vi "removeNode2.vi"(0 "reference":refnum<class "Graph.lvclass">, 1 "node":refnum<class "AbstractNode.lvclass">, 5 "error in (no error)":errorcluster) -> (14 "reference out":refnum<class "Graph.lvclass">, 19 "error out":errorcluster)   [LabVIEW 2016, in "Graph.lvclass"]
uses:
  <resource>/Framework/Providers/Open_GDS/UML/Graph_class/Graph.lvclass
  <resource>/Framework/Providers/Open_GDS/UML/AbstractNode_class/AbstractNode.lvclass
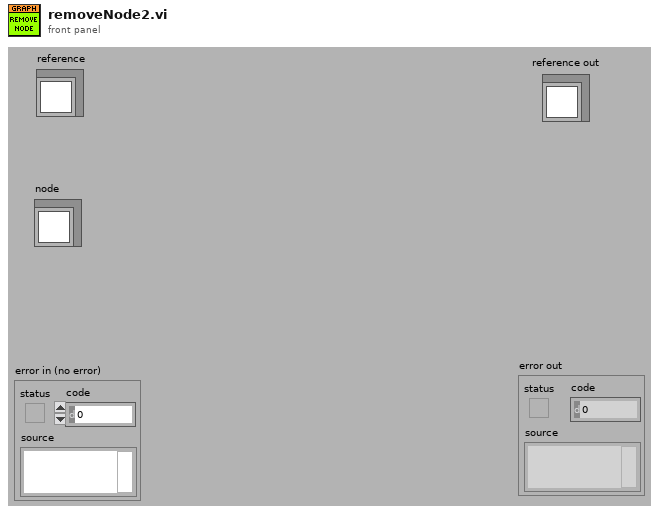
[diagram p1: front panel]
types:
  T1 = typedef "Graph.lvclass/ObjectAttributes.ctl" = cluster{"nodes":refnum<class "AbstractNode.lvclass">[], "edges":refnum<class "AbstractEdge.lvclass">[], "nodesToBeRemoved":refnum<class "AbstractNode.lvclass">[], "edgesToBeRemoved":refnum<class "AbstractEdge.lvclass">[], "needsLayout":bool, "LayoutNodes":refnum<class "AbstractNode.lvclass">[]}
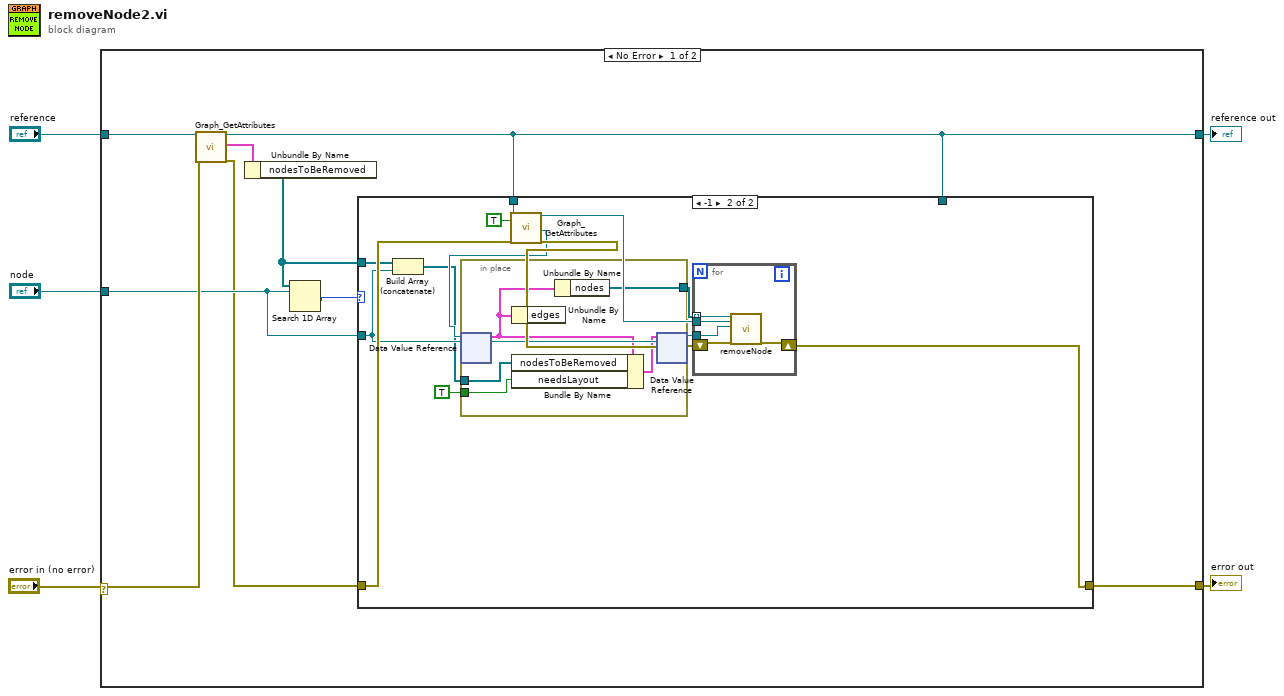
[diagram p0: block diagram]
diagram:
  n1 = case shown="No Error" "error in (no error)" {
    selector: "error in (no error)" -> [w11 w38]
    tunnel: "reference" -> [w14 w39]
    tunnel: [w13 w38] -> w4
    tunnel: [w12 w39] -> w3
    tunnel: "node" -> [w10 _]
    frame No Error {
      n2 = call <resource>:"Graph_GetAttributes.vi"("reference in"=w14, "error in (no error)"=w11) -> ("reference out"=w12:refnum<class "Graph.lvclass">, "Data"=w6:T1, "error out"=w8:errorcluster)  [unwired: 1 in, 14 out]
      n3 = Unbundle By Name(w6) -> ("nodesToBeRemoved"=w7:refnum<class "AbstractNode.lvclass">[])
      n4 = Search 1D Array(1D array=w7, element=w10) -> (index of element=w9:i32)  [unwired: 1 out]
      n5 = case shown="-1" w9 {
        tunnel: w8 -> [w15 w26]
        tunnel: [w15 w21] -> w13
        tunnel: w12 -> [_ w27]
        tunnel: w7 -> [_ w25]
        tunnel: w10 -> [_ w22]
        tunnel: w12 -> [_ _]
        frame 0, Default {
        }
        frame -1 {
          n6 = Build Array (concatenate)(w25, w22) -> (w17:refnum<class "AbstractNode.lvclass">[])
          n7 = call <resource>:"Graph_GetAttributes.vi"("reference in"=w27, "OnlyGetDvrReference(False)"=TRUE, "error in (no error)"=w26) -> ("reference out"=w24:refnum<class "Graph.lvclass">, "DataRef"=w19:refnum<data-value>, "error out"=w23:errorcluster)  [unwired: 13 in, 1 out]
          n8 = in-place {
            in-place-border: [w31] -> w18
            in-place-border: w17 -> [w30]
            in-place-border: TRUE ("needsLayout") -> [w29]
            n9 = in-place-dvr #1(w19) -> (w32:T1)  [unwired: 1 out]
            n10 = Unbundle By Name(w32) -> ()  [unwired: 1 out]
            n11 = Bundle By Name(cluster=w32, "nodesToBeRemoved"=w30, "needsLayout"=w29) -> (w28:T1)
            n12 = Unbundle By Name(w32) -> ("nodes"=w31:refnum<class "AbstractNode.lvclass">[])
            n13 = in-place-dvr #1(w28) -> ()  [unwired: 2 out]
          }
          n14 = for {
            tunnel: w18 -> [w37] mode=indexing
            tunnel: w24 -> [w36]
            tunnel: w22 -> [w35]
            shift-right: [w33] -> w21
            shift-left: w23 -> [w34]
            n15 = call-dynamic "removeNode.vi"("reference"=w37, "graph"=w36, "node"=w35, "error in (no error)"=w34) -> ("error out"=w33:errorcluster)  [unwired: 14 in, 1 out]
          }
        }
      }
    }
    frame Error {
    }
  }
  "reference out" <- w3
  "error out" <- w4
